vi "AnalogTrack.vi"(0 "controller":refnum<k24>, 1 "axis name":string, 2 "analog output":i32, 3 "servo value":i32, 4 "scale factor":dbl=1.0, 5 "error in (no error)":errorcluster, 6 "offset value":dbl, 7 "return immediately":bool, 8 "min value":dbl, 9 "taskId":i32(ring) items=["TLibrary", "T01", "T02", "T03", "T04", "T05", "T06", "T07", "T08", "T09", "T10", "T11", "T12", "T13", "T14", "T15", "T16", "T17", "T18", "T19", "T20", "T21", "T22", "T23", "T24", "T25", "T26", "T27", "T28", "T29", "T30", "T31"], 10 "max value":dbl) -> (14 "controller out":refnum<k24>, 19 "error out":errorcluster)   [LabVIEW 2016, in "Aerotech VIs.lvlib"]
uses:
  Aerotech VIs.lvlib
  C:/Users/HEP Gantry/Documents/Assembly/V4/Drivers/Aerotech A3200/Bin/Aerotech.A3200.dll
  V4/Drivers/Aerotech A3200/Bin/Aerotech.A3200.dll
  C:/Users/HEP Gantry/Documents/Assembly/V4/Drivers/Aerotech A3200/Bin/Aerotech.A3200.LabVIEW.dll
  V4/Drivers/Aerotech A3200/Bin/Aerotech.A3200.LabVIEW.dll
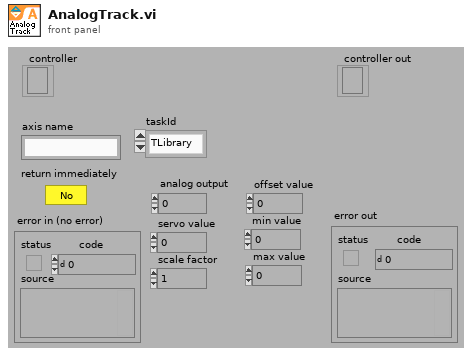
[diagram p1: front panel]
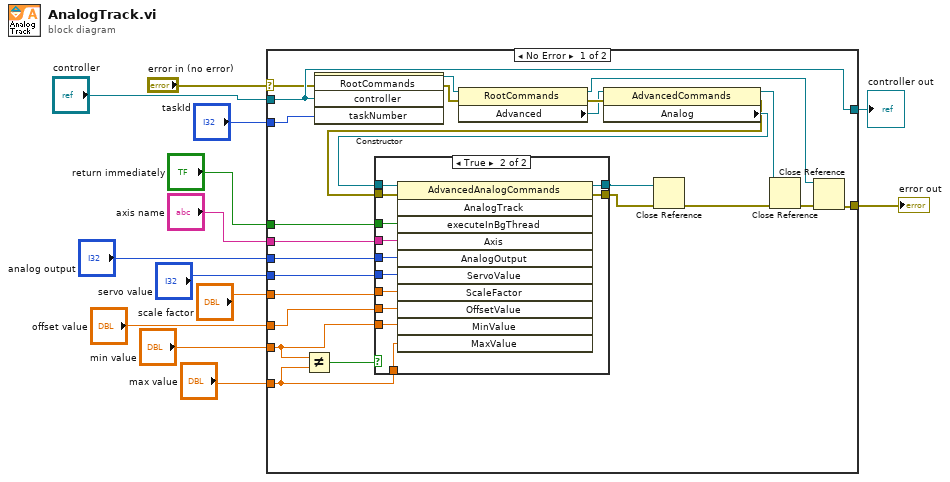
[diagram p0: block diagram]
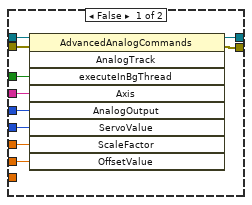
[diagram p2: hidden frame]
diagram:
  n1 = case shown="No Error" "error in (no error)" {
    selector: "error in (no error)" -> [w33 w62]
    tunnel: [w38 w62] -> w12
    tunnel: "controller" -> [w34 w61]
    tunnel: "return immediately" -> [w24 _]
    tunnel: "axis name" -> [w23 _]
    tunnel: "analog output" -> [w22 _]
    tunnel: [w34 w61] -> w1
    tunnel: "servo value" -> [w21 _]
    tunnel: "scale factor" -> [w20 _]
    tunnel: "offset value" -> [w19 _]
    tunnel: "min value" -> [w17 _]
    tunnel: "max value" -> [w16 _]
    tunnel: "taskId" -> [w27 _]
    frame No Error {
      n2 = Not Equal?(x=w17, y=w16) -> (x != y?=w18:bool)
      n3 = constructor class="RootCommands"(error in=w33, "controller"=w34, "taskNumber"=w27) -> (reference out=w29:refnum<k24>, error out=w28:errorcluster)  [unwired: 2 in, 3 out]
      n4 = property class="RootCommands"(reference=w29, error in=w28) -> (reference out=w31:refnum<k24>, error out=w32:errorcluster, "Advanced"=w30:refnum<k24>)
      n5 = property class="AdvancedCommands"(reference=w30, error in=w32) -> (reference out=w36:refnum<k24>, error out=w25:errorcluster, "Analog"=w26:refnum<k24>)
      n6 = case shown="True" w18 {
        tunnel: w26 -> [w48 w58]
        tunnel: w25 -> [w47 w57]
        tunnel: w24 -> [w46 w51]
        tunnel: w23 -> [w45 w52]
        tunnel: w22 -> [w44 w53]
        tunnel: [w43 w59] -> w14
        tunnel: [w42 w60] -> w15
        tunnel: w21 -> [w41 w54]
        tunnel: w20 -> [w40 w55]
        tunnel: w19 -> [w39 w56]
        tunnel: w16 -> [_ w49]
        tunnel: w17 -> [_ w50]
        frame False {
          n7 = invoke class="AdvancedAnalogCommands" method="AnalogTrack"(reference=w48, error in=w47, "executeInBgThread"=w46, "Axis"=w45, "AnalogOutput"=w44, "ServoValue"=w41, "ScaleFactor"=w40, "OffsetValue"=w39) -> (reference out=w42:refnum<k24>, error out=w43:errorcluster)  [unwired: 1 in, 7 out]
        }
        frame True {
          n8 = invoke class="AdvancedAnalogCommands" method="AnalogTrack"(reference=w58, error in=w57, "executeInBgThread"=w51, "Axis"=w52, "AnalogOutput"=w53, "ServoValue"=w54, "ScaleFactor"=w55, "OffsetValue"=w56, "MinValue"=w50, "MaxValue"=w49) -> (reference out=w60:refnum<k24>, error out=w59:errorcluster)  [unwired: 1 in, 9 out]
        }
      }
      n9 = Close Reference(reference=w15, error in (no error)=w14) -> (error out=w35:errorcluster)
      n10 = Close Reference(reference=w36, error in (no error)=w35) -> (error out=w37:errorcluster)
      n11 = Close Reference(reference=w31, error in (no error)=w37) -> (error out=w38:errorcluster)
    }
    frame Error {
    }
  }
  "error out" <- w12
  "controller out" <- w1
